vi "CTR_DAQNodeConfigs.vi"(8 "error in":errorcluster, 10 "StreamCluster_TypeDef in":T1={"DAQ_Configs"=[], "CTR_Config"={"CTR refDes"="", "CTR IP Addr"=""}, "Network_Configs"={"Buffer"=1, "ManagmentRate_Hz"=1000, "StreamRate_Hz"=10, "ConnectionHysterisis"=0, "LoggingRate_Hz"=10}, "ConfigXML_Checksum"=""}, 11 "DOM document in":refnum<k20>) -> (0 "error out":errorcluster={"status"=TRUE, "code"=-2633, "source"="Property Node (arg 1) in NI_XML.lvlib:Get Node Text Content.vi->CTR_ControlNodeConfigs.vi->CTR_ReadXML_Config.vi->CTRnode.vi"}, 2 "StreamCluster_TypeDef out":T1={"DAQ_Configs"=[], "CTR_Config"={"CTR refDes"="", "CTR IP Addr"=""}, "Network_Configs"={"Buffer"=1, "ManagmentRate_Hz"=1000, "StreamRate_Hz"=10, "ConnectionHysterisis"=0, "LoggingRate_Hz"=10}, "ConfigXML_Checksum"=""}, 3 "DOM document out":refnum<k20>)   [LabVIEW 2024]
uses:
  Control/StreamCluster_TypeDef.ctl
  Control/streamIO_states.ctl
  <vilib>/xml/Close Reference(Node).vi
  <vilib>/Utility/error.llb/Error Cluster From Error Code.vi
  <vilib>/ErrorRing/Error Ring.xnode
  <vilib>/xml/NI_XML.lvlib
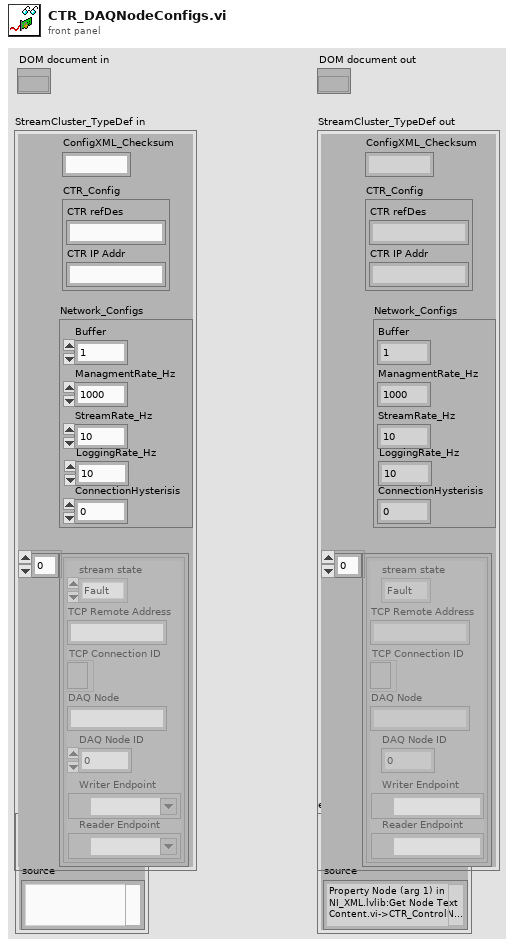
[diagram p1: front panel]
types:
  T1 = typedef "StreamCluster_TypeDef.ctl" = cluster{"DAQ_Configs":cluster{"stream state":T2, "TCP Remote Address":string, "TCP Connection ID":refnum<k5>, "DAQ Node":string, "DAQ Node ID":i32, "Writer Endpoint":refnum<k21>, "Reader Endpoint":refnum<k21>}[], "CTR_Config":cluster{"CTR refDes":string, "CTR IP Addr":string}, "Network_Configs":cluster{"Buffer":i32, "ManagmentRate_Hz":i32, "StreamRate_Hz":i32, "ConnectionHysterisis":i32, "LoggingRate_Hz":i32}, "ConfigXML_Checksum":string}
  T2 = typedef "streamIO_states.ctl" = enum16{"Fault", "Initialize", "Stream", "Close"}
  T3 = cluster{"[0]":string, "[1]":string, "[2]":string, "[3]":string, "[4]":string, "[5]":string, "[6]":string, "[7]":string, "[8]":string}
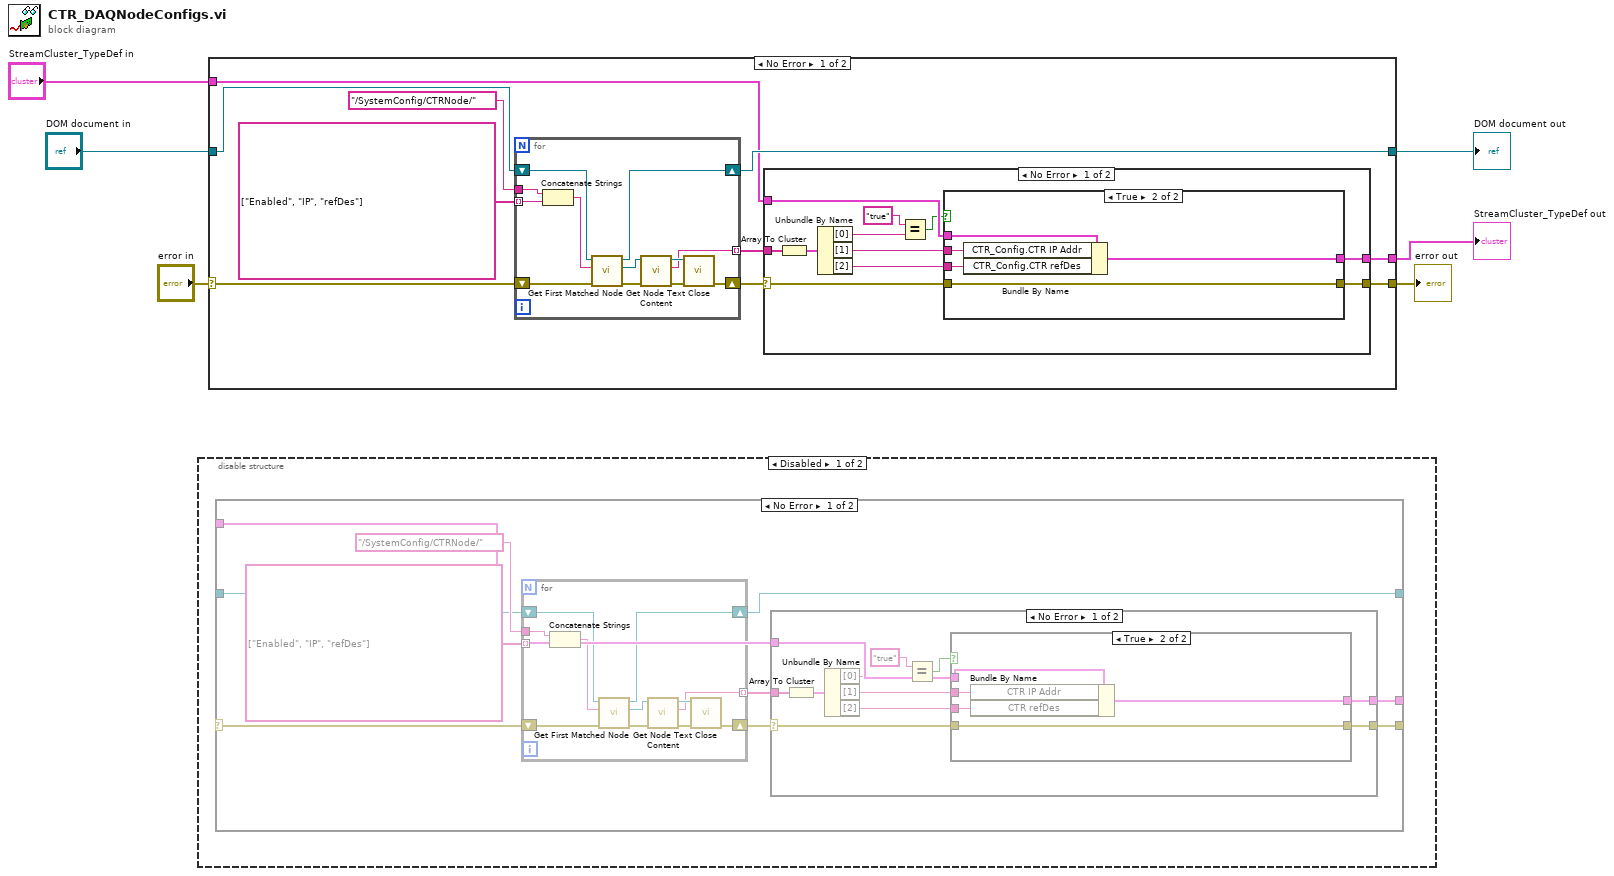
[diagram p0: block diagram]
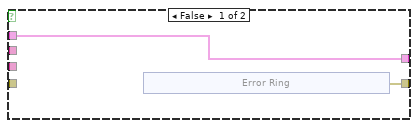
[diagram p2: hidden frame]
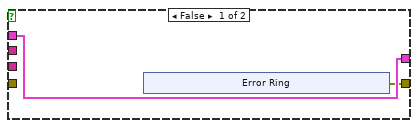
[diagram p6: hidden frame]
diagram:
  n1 = disable-structure shown="Disabled" {
    frame Disabled {
      n2 = case shown="No Error" {
        selector: _ -> [w16 w56]
        tunnel: [w8 w56] -> _
        tunnel: _ -> [w14 w54]
        tunnel: [w12 w54] -> _
        tunnel: _ -> [w10 w55]
        tunnel: [w9 w55] -> _
        frame No Error {
          n3 = for {
            tunnel: "/SystemConfig/CTRNode/" ("XPath expression") -> [w49]
            tunnel: string[] ["Enabled", "IP", "refDes"] -> [w48] mode=indexing
            shift-right: [w44] -> w12
            shift-left: w14 -> [w50]
            shift-right: [w43] -> w7
            shift-left: w16 -> [w51]
            tunnel: [w42] -> w11 mode=indexing
            n4 = Concatenate Strings(w49, w48) -> (w47:string)
            n5 = call <vilib>:"Get First Matched Node.vi"("error in (no error)"=w51, "XPath expression"=w47, "node in"=w50) -> ("error out"=w52:errorcluster, "node result"=w53:refnum<k20>, "node out"=w44:refnum<k20>)  [unwired: 6 in]
            n6 = call <vilib>:"Get Node Text Content.vi"("error in (no error)"=w52, "node in"=w53) -> ("error out"=w46:errorcluster, "node text"=w42:string, "node out"=w45:refnum<k20>)  [unwired: 7 in]
            n7 = call-poly <vilib>:"Close.vi"("error in (no error)"=w46, "node"=w45) -> ("error out"=w43:errorcluster)  [unwired: 7 out]
          }
          n8 = case shown="No Error" w7 {
            selector: w7 -> [w17 w41]
            tunnel: w11 -> [w27 _]
            tunnel: w10 -> [w25 w40]
            tunnel: [w24 w40] -> w9
            tunnel: [w18 w41] -> w8
            frame No Error {
              n9 = Array To Cluster(array=w27) -> (cluster=w26:T3)
              n10 = Unbundle By Name(w26) -> ("[0]"=w23:string, "[1]"=w20:string, "[2]"=w19:string)
              n11 = Equal?(x="true", y=w23) -> (x = y?=w21:bool)
              n12 = case shown="True" w21 {
                tunnel: w25 -> [w29 w39]
                tunnel: [w29 w38] -> w24
                tunnel: w20 -> [_ w37]
                tunnel: w19 -> [_ w36]
                tunnel: w17 -> [_ w35]
                tunnel: [w28 w35] -> w18
                frame False {
                  n13 = xnode "Error Ring"() -> ("error out"=w28:errorcluster)
                }
                frame True {
                  n14 = Bundle By Name(cluster=w39, "CTR IP Addr"=w37, "CTR refDes"=w36) -> (w38:cluster{})
                }
              }
            }
            frame Error {
            }
          }
        }
        frame Error {
        }
      }
    }
    frame Enabled {
    }
  }
  n15 = case shown="No Error" "error in" {
    selector: "error in" -> [w66 w106]
    tunnel: [w58 w106] -> w5
    tunnel: "DOM document in" -> [w64 w104]
    tunnel: [w62 w104] -> w3
    tunnel: "StreamCluster_TypeDef in" -> [w60 w105]
    tunnel: [w59 w105] -> w1
    frame No Error {
      n16 = for {
        tunnel: "/SystemConfig/CTRNode/" ("XPath expression") -> [w99]
        tunnel: string[] ["Enabled", "IP", "refDes"] -> [w98] mode=indexing
        shift-right: [w94] -> w62
        shift-left: w64 -> [w100]
        shift-right: [w93] -> w57
        shift-left: w66 -> [w101]
        tunnel: [w92] -> w61 mode=indexing
        n17 = Concatenate Strings(w99, w98) -> (w97:string)
        n18 = call <vilib>:"Get First Matched Node.vi"("error in (no error)"=w101, "XPath expression"=w97, "node in"=w100) -> ("error out"=w102:errorcluster, "node result"=w103:refnum<k20>, "node out"=w94:refnum<k20>)  [unwired: 6 in]
        n19 = call <vilib>:"Get Node Text Content.vi"("error in (no error)"=w102, "node in"=w103) -> ("error out"=w96:errorcluster, "node text"=w92:string, "node out"=w95:refnum<k20>)  [unwired: 7 in]
        n20 = call-poly <vilib>:"Close.vi"("error in (no error)"=w96, "node"=w95) -> ("error out"=w93:errorcluster)  [unwired: 7 out]
      }
      n21 = case shown="No Error" w57 {
        selector: w57 -> [w67 w91]
        tunnel: w61 -> [w77 _]
        tunnel: w60 -> [w75 w90]
        tunnel: [w74 w90] -> w59
        tunnel: [w68 w91] -> w58
        frame No Error {
          n22 = Array To Cluster(array=w77) -> (cluster=w76:T3)
          n23 = Unbundle By Name(w76) -> ("[0]"=w73:string, "[1]"=w70:string, "[2]"=w69:string)
          n24 = Equal?(x="true", y=w73) -> (x = y?=w71:bool)
          n25 = case shown="True" w71 {
            tunnel: w75 -> [w79 w89]
            tunnel: [w79 w88] -> w74
            tunnel: w70 -> [_ w87]
            tunnel: w69 -> [_ w86]
            tunnel: w67 -> [_ w85]
            tunnel: [w78 w85] -> w68
            frame False {
              n26 = xnode "Error Ring"() -> ("error out"=w78:errorcluster)
            }
            frame True {
              n27 = Bundle By Name(cluster=w89, "CTR_Config.CTR IP Addr"=w87, "CTR_Config.CTR refDes"=w86) -> (w88:T1)
            }
          }
        }
        frame Error {
        }
      }
    }
    frame Error {
    }
  }
  "error out" <- w5
  "DOM document out" <- w3
  "StreamCluster_TypeDef out" <- w1
